vi "0main.vi"   [LabVIEW 2022 SP3]
panel:
  # "PRESS RUN TO START"
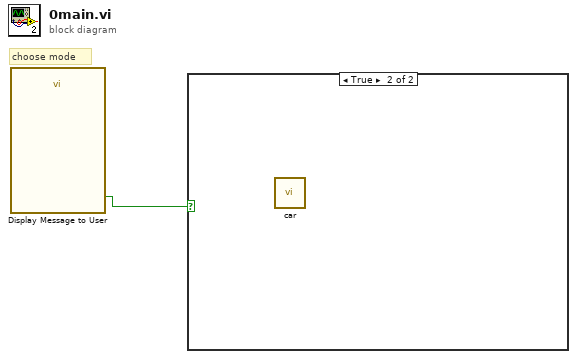
[diagram p0: block diagram]
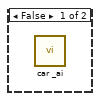
[diagram p2: hidden frame]
diagram:
  # "choose mode"
  n1 = call "Display Message to User"() -> ("Real Player"=w1:bool)  [unwired: 10 in, 1 out]
  n2 = case shown="True" w1 {
    frame False {
      n3 = call "car _ai.vi"() -> ()  [unwired: 12 in]
    }
    frame True {
      n4 = call "car.vi"() -> ()  [unwired: 12 in]
    }
  }
